vi "ziModSetValueBinary.vi"(8 "Error In":errorcluster, 9 "Data":string, 10 "Path":string, 11 "ModHandle In":T1 {"ModHandle" format="0x%08x"; "Conn" format="0x%08x"}) -> (0 "Error Out":errorcluster, 3 "ModHandle Out":T1 {"ModHandle" format="0x%08x"; "Conn" format="0x%08x"})   [LabVIEW 2015, in "Zurich Instruments LabOne.lvlib"]
doc: "This vi writes the string as bytes of binary data to the <b>module</b> nodes specified by <b>Path</b>."
uses:
  Zurich Instruments LabOne.lvlib
  Zurich Instruments/LabOne/API/LabVIEW/Zurich Instruments LabOne/Private/ziLV64.framework
  ziTypeModHandle.ctl
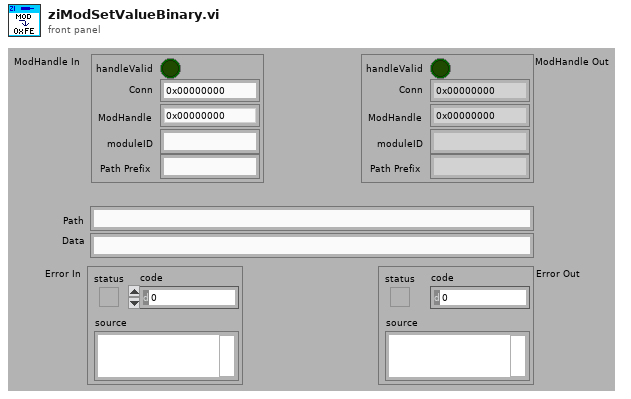
[diagram p1: front panel]
types:
  T1 = typedef "Zurich Instruments LabOne.lvlib/ziTypeModHandle.ctl" = cluster{"handleValid":bool, "Conn":u64, "ModHandle":u64, "moduleID":string, "Path Prefix":string}
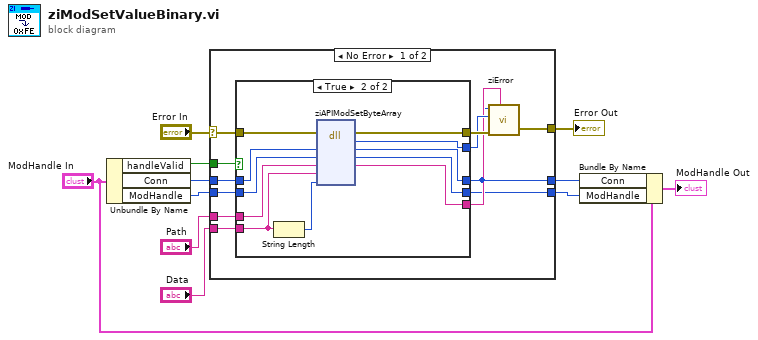
[diagram p0: block diagram]
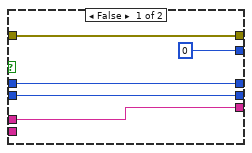
[diagram p2: hidden frame]
diagram:
  n1 = Unbundle By Name("ModHandle In") -> ("handleValid"=w1:bool, "Conn"=w3:u64, "ModHandle"=w5:u64)
  n2 = case shown="No Error" "Error In" {
    selector: "Error In" -> [w18 w42]
    tunnel: "Data" -> [w23 _]
    tunnel: [w22 w42] -> w10
    tunnel: "Path" -> [w15 _]
    tunnel: w5 -> [w17 w41]
    tunnel: [w16 w41] -> w4
    tunnel: w3 -> [w14 w40]
    tunnel: [w12 w40] -> w2
    tunnel: w1 -> [w13 _]
    frame No Error {
      n3 = case shown="True" w13 {
        tunnel: w18 -> [w28 w39]
        tunnel: w15 -> [w26 w38]
        tunnel: w23 -> [_ w33]
        tunnel: [w28 w37] -> w21
        tunnel: [u32 0 ("return type") w36] -> w20
        tunnel: [w24 w35] -> w12
        tunnel: [w26 w34] -> w19
        tunnel: w17 -> [w25 w31]
        tunnel: [w25 w30] -> w16
        tunnel: w14 -> [w24 w29]
        frame False {
        }
        frame True {
          n4 = String Length(string=w33) -> (length=w32:i32)
          n5 = dll-call lib="Users/arkady/Desktop/ado/github/resonant_ultrasound_arxiv/maglab ultrasound -- arkady --arxiv/Zurich Instruments/LabOne/API/LabVIEW/Zurich Instruments LabOne/Private/ziLV*.*" fn="ziAPIModSetByteArray"(error in=w39, "Conn"=w29, "ModHandle"=w31, "Path"=w38, "Value"=w33, "Len"=w32) -> (error out=w37:errorcluster, "return type"=w36:u32, "Conn"=w35:u64, "ModHandle"=w30:u64, "Path"=w34:string)  [unwired: 4 in, 1 out]
        }
      }
      n6 = call "ziError.vi"("Conn"=w12, "ziErrorCode"=w20, "Error In"=w21, "Annotation"=w19) -> ("Error Out"=w22:errorcluster)  [unwired: 1 in, 1 out]
    }
    frame Error {
    }
  }
  "Error Out" <- w10
  n7 = Bundle By Name(cluster="ModHandle In", "Conn"=w2, "ModHandle"=w4) -> (→"ModHandle Out":T1)
